vi "Correct_Position_info for 2nd FFID with rotation.vi"() -> (0 "error out":errorcluster, 4 "Path":path)   [LabVIEW 2017]
panel:
  in  "Offset Position":sgl[](array[numeric])
  out "File Changed":bool
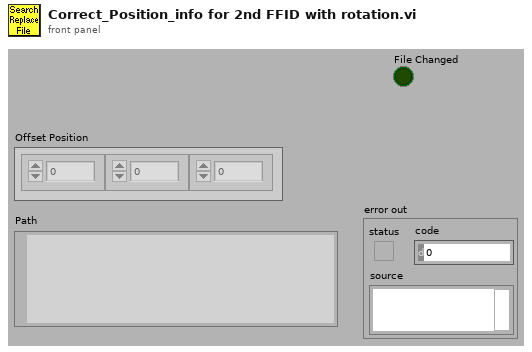
[diagram p1: front panel]
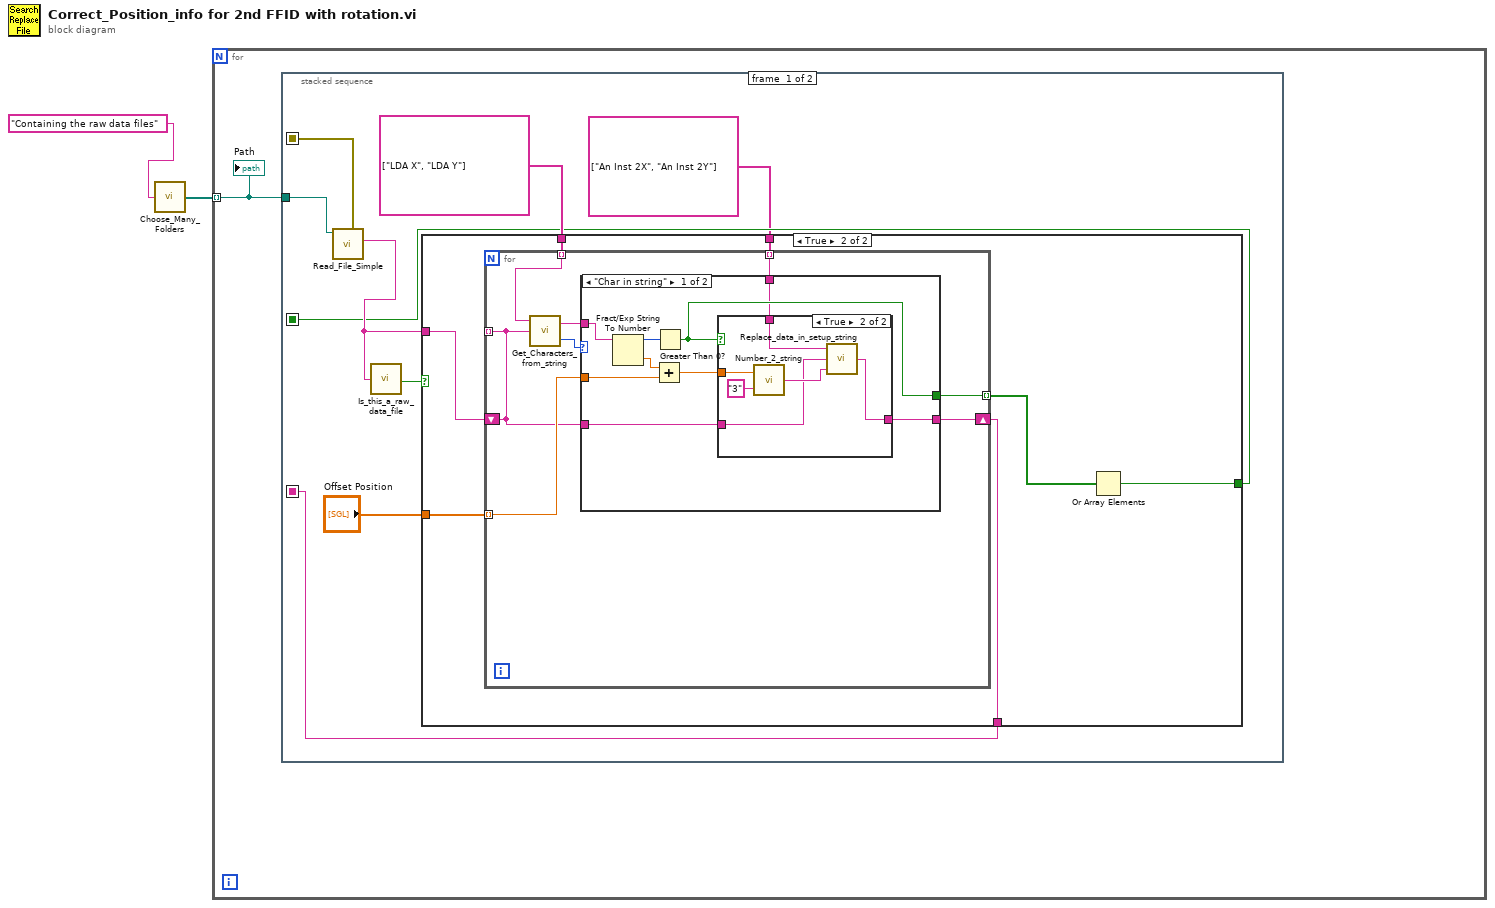
[diagram p0: block diagram]
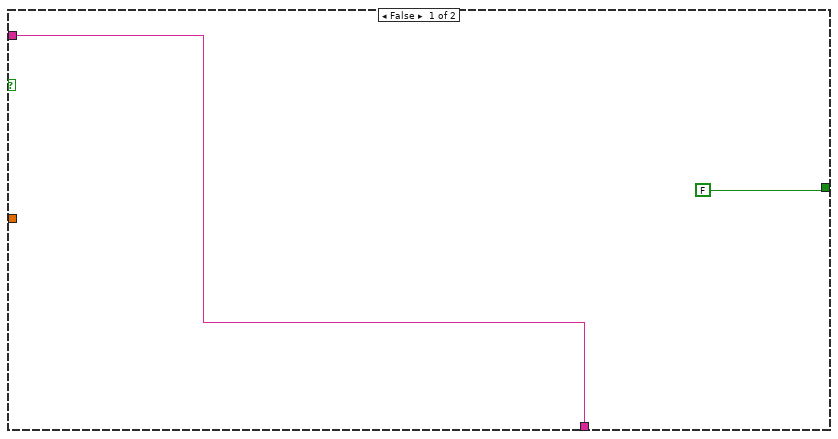
[diagram p2: hidden frame]
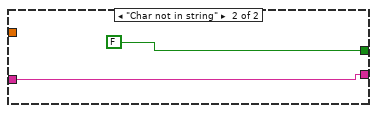
[diagram p4: hidden frame]
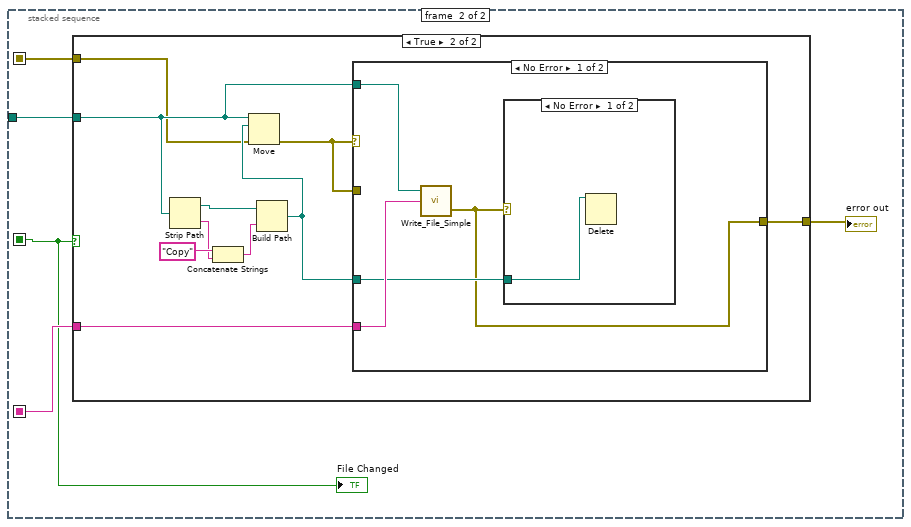
[diagram p5: hidden frame]
diagram:
  n1 = call "Choose_Many_Folders.vi"("Purpose of choosing folder"="Containing the raw data files") -> ("Files"=w1:path[])
  n2 = for {
    tunnel: w1 -> [w3] mode=indexing
    n3 = stacked-sequence {
      seq-local: [w11 _] -> [_ w49]
      seq-local: [w5 _] -> [_ w50]
      seq-local: [w6 _] -> [_ w48]
      tunnel: w3 -> [w12 w52]
      frame #0 {
        n4 = call "Read_File_Simple.vi"("Filename"=w12) -> ("error out"=w11:errorcluster, "string"=w8:string)  [unwired: 4 in, 4 out]
        n5 = call "Is_this_a_raw_data_file.vi"("character string"=w8) -> ("Raw Dat File?"=w10:bool)  [unwired: 2 out]
        n6 = case shown="True" w10 {
          tunnel: string[] ["LDA X", "LDA Y"] -> [_ w21]
          tunnel: [FALSE w16] -> w6
          tunnel: w8 -> [w13 w18]
          tunnel: "Offset Position" -> [_ w19]
          tunnel: [w13 w17] -> w5
          tunnel: string[] ["An Inst 2X", "An Inst 2Y"] -> [_ w15]
          frame False {
          }
          frame True {
            n7 = for {
              tunnel: w21 -> [w25] mode=indexing
              tunnel: [w27] -> w20 mode=indexing
              tunnel: [w24] -> _ mode=indexing
              tunnel: w19 -> [w26] mode=indexing
              shift-right: [w23] -> w17
              shift-left: w18 -> [w24]
              tunnel: w15 -> [w22] mode=indexing
              n8 = call "Get_Characters_from_string.vi"("Input string"=w24, "Variable name"=w25) -> ("Status"=w28:enum16{"Char in string", "Char not in string"}, "Value"=w29:string)  [unwired: 1 in]
              n9 = case shown="\"Char in string\"" w28 {
                tunnel: w29 -> [w38 _]
                tunnel: [w31 FALSE] -> w27
                tunnel: w26 -> [w36 _]
                tunnel: w24 -> [w33 w46]
                tunnel: [w32 w46] -> w23
                tunnel: w22 -> [w30 _]
                frame "Char in string" {
                  n10 = Fract/Exp String To Number(string=w38) -> (offset past number=w35:i32, number=w37:dbl)  [unwired: 3 in]
                  n11 = Add(x=w37, y=w36) -> (x+y=w34:dbl)
                  n12 = Greater Than 0?(x=w35) -> (x > 0?=w31:bool)
                  n13 = case shown="True" w31 {
                    tunnel: w34 -> [_ w45]
                    tunnel: w30 -> [_ w42]
                    tunnel: w33 -> [w39 w41]
                    tunnel: [w39 w40] -> w32
                    frame False {
                    }
                    frame True {
                      n14 = call "Number_2_string.vi"("precision"="3", "number"=w45) -> ("String"=w43:string)
                      n15 = call "Replace_data_in_setup_string.vi"("New data string"=w43, "Input string"=w41, "Variable name"=w42) -> ("Appended string"=w40:string)
                    }
                  }
                }
                frame "Char not in string" {
                }
              }
            }
            n16 = Or Array Elements(Boolean array=w20) -> (logical OR=w16:bool)
          }
        }
      }
      frame #1 {
        n17 = case shown="True" w48 {
          tunnel: w52 -> [_ w59]
          tunnel: w50 -> [_ w58]
          tunnel: [w53 w56] -> w51
          tunnel: w49 -> [w53 w54]
          frame False {
          }
          frame True {
            n18 = Strip Path(path=w59) -> (stripped path=w60:path, name=w62:string)
            n19 = Concatenate Strings("Copy" ("name or relative path"), w62) -> (w61:string)
            n20 = Build Path(base path=w60, name or relative path=w61) -> (appended path=w57:path)
            n21 = Move(source path=w59, error in=w54, 10:w57) -> (error out=w55:errorcluster)  [unwired: 2 in, 2 out]
            n22 = case shown="No Error" w55 {
              tunnel: w59 -> [w67 _]
              tunnel: w58 -> [w66 _]
              tunnel: w57 -> [w65 _]
              tunnel: [w64 w69] -> w56
              tunnel: w55 -> [_ w69]
              frame No Error {
                n23 = call "Write_File_Simple.vi"("character string"=w66, "file path"=w67) -> ("error out"=w64:errorcluster)  [unwired: 1 in, 1 out]
                n24 = case shown="No Error" w64 {
                  tunnel: w65 -> [w68 _]
                  frame No Error {
                    n25 = Delete(path (use dialog)=w68) -> ()  [unwired: 4 in, 3 out]
                  }
                  frame Error {
                  }
                }
              }
              frame Error {
              }
            }
          }
        }
        "error out" <- w51
        "File Changed" <- w48
      }
    }
    "Path" <- w3
  }
